vi "data to registers.vi"(9 "specifications":T1[](array[typedef]), 10 "allocation":u16[](array[numeric]), 11 "data table":T3) -> (2 "registers":u16[](array[numeric]), 3 "allocation":T3)   [LabVIEW 2013, in "Modbus Slave runtime.lvclass"]
uses:
  Modbus Slave runtime.lvclass
  <vilib>/NI/Tag Bus/table/data table.ctl
  data mapping elements.ctl
  <vilib>/NI/Tag Bus/tag/Data Type.ctl
  <vilib>/NI/Tag Bus/table/data polymorphs/read one/read Double.vi
  <vilib>/NI/Tag Bus/table/data polymorphs/read one/read Single.vi
  <vilib>/NI/Tag Bus/table/data polymorphs/read one/read I64.vi
  <vilib>/NI/Tag Bus/table/data polymorphs/read one/read U64.vi
  <vilib>/NI/Tag Bus/table/data polymorphs/read one/read I32.vi
  <vilib>/NI/Tag Bus/table/data polymorphs/read one/read U32.vi
  <vilib>/NI/Tag Bus/table/data polymorphs/read one/read I16.vi
  <vilib>/NI/Tag Bus/table/data polymorphs/read one/read U16.vi
  <vilib>/NI/Tag Bus/table/data polymorphs/read one/read I8.vi
  <vilib>/NI/Tag Bus/table/data polymorphs/read one/read U8.vi
  <vilib>/NI/Tag Bus/table/data polymorphs/read one/read Boolean.vi
  <vilib>/NI/Tag Bus/table/data table.lvlib
  <vilib>/NI/Tag Bus/tag/tag descriptor.lvclass
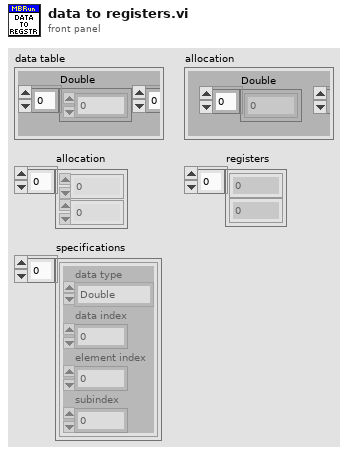
[diagram p1: front panel]
types:
  T1 = typedef "Modbus Slave runtime.lvclass/data mapping elements.ctl" = cluster{"data type":T2, "data index":i32, "element index":i32, "subindex":i32}
  T2 = typedef "tag bus.lvlib/tag descriptor.lvclass/Data Type.ctl" = enum16{"Double", "Single", "I64", "I32", "I16", "I8", "U64", "U32", "U16", "U8", "Boolean", "String", "Array of Double", "Array of Single", "Array of I64", "Array of I32", "Array of I16", "Array of I8", "Array of U64", "Array of U32", "Array of U16", "Array of U8", "Array of Boolean", "Array of String"}
  T3 = typedef "tag bus.lvlib/data table.lvlib/data table.ctl" = cluster{"Double":dbl[], "Single":sgl[], "I64":i64[], "I32":i32[], "I16":i16[], "I8":i8[], "U64":u64[], "U32":u32[], "U16":u16[], "U8":u8[], "Boolean":bool[], "String":string[], "Array of Double":cluster{"DBL Array":dbl[]}[], "Array of Single":cluster{"SGL Array":sgl[]}[], "Array of I64":cluster{"I64 Array":i64[]}[], "Array of I32":cluster{"I32 Array":i32[]}[], "Array of I16":cluster{"I16 Array":i16[]}[], "Array of I8":cluster{"I8 Array":i8[]}[], "Array of U64":cluster{"U64 Array":u64[]}[], "Array of U32":cluster{"U32 Array":u32[]}[], "Array of U16":cluster{"U16 Array":u16[]}[], "Array of U8":cluster{"U8 Array":u8[]}[], "Array of Boolean":cluster{"Boolean Array":bool[]}[], "Array of String":cluster{"String Array":string[]}[]}
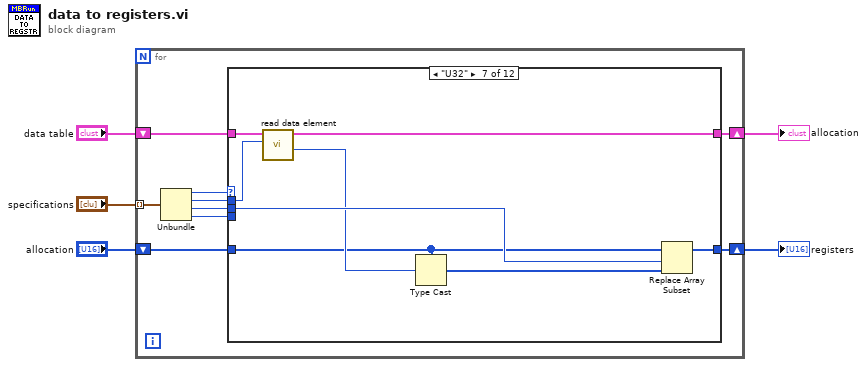
[diagram p0: block diagram]
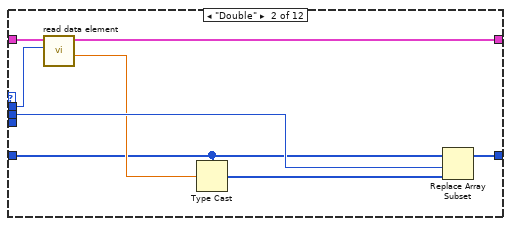
[diagram p3: hidden frame]
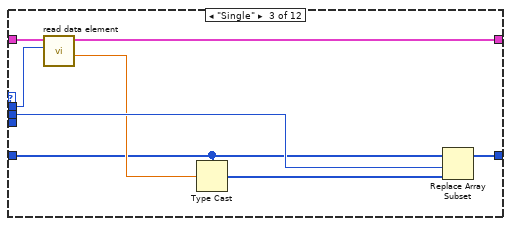
[diagram p4: hidden frame]
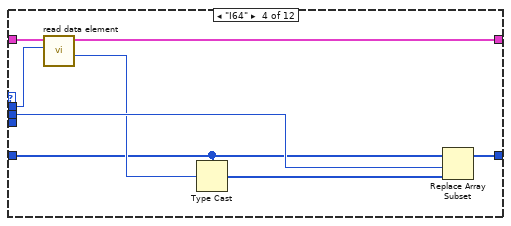
[diagram p5: hidden frame]
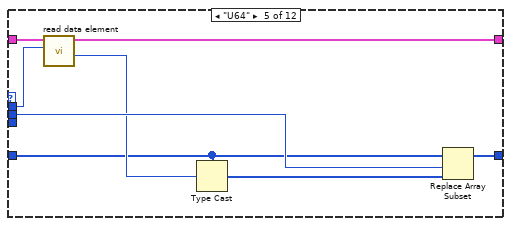
[diagram p6: hidden frame]
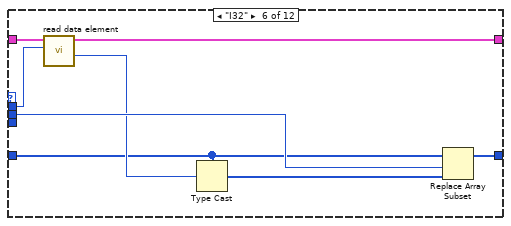
[diagram p7: hidden frame]
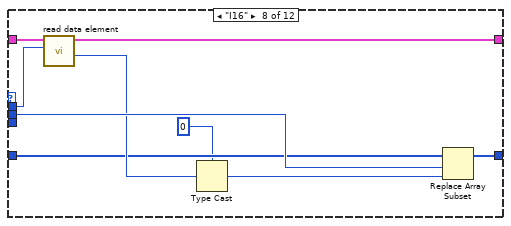
[diagram p8: hidden frame]
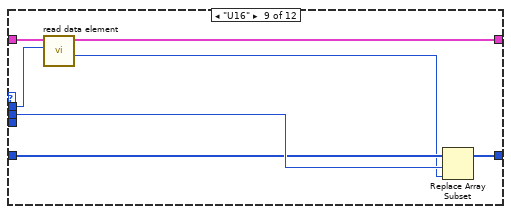
[diagram p9: hidden frame]
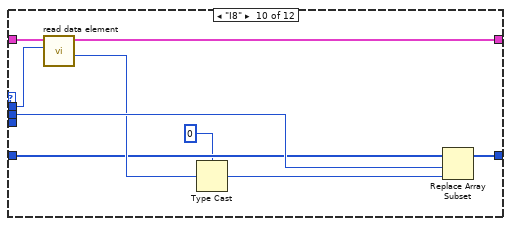
[diagram p10: hidden frame]
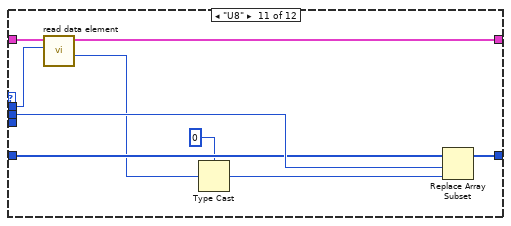
[diagram p11: hidden frame]
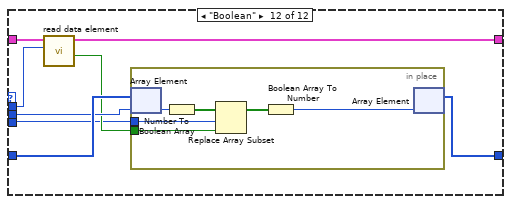
[diagram p12: hidden frame]
diagram:
  n1 = for {
    shift-right: [w11] -> w4
    shift-left: "data table" -> [w12]
    tunnel: "specifications" -> [w14] mode=indexing
    shift-right: [w7] -> w1
    shift-left: "allocation" -> [w10]
    n2 = Unbundle(w14) -> ("data type"=w13:T2, "data index"=w9:i32, "element index"=w6:i32, "subindex"=w8:i32)
    n3 = case shown="\"U32\"" w13 {
      tunnel: w12 -> [w16 w24 w32 w40 w48 w56 w64 w73 w80 w89 w98 w106]
      tunnel: [w16 w23 w31 w39 w47 w55 w63 w72 w79 w88 w97 w105] -> w11
      tunnel: w6 -> [_ w20 w28 w36 w44 w52 w60 w69 w76 w85 w94 w101]
      tunnel: w10 -> [w15 w18 w26 w34 w42 w50 w58 w67 w75 w83 w93 w103]
      tunnel: w9 -> [_ w22 w30 w38 w46 w54 w62 w71 w78 w87 w96 w104]
      tunnel: w8 -> [_ _ _ _ _ _ _ _ _ _ _ w99]
      tunnel: [w15 w21 w29 w37 w45 w53 w61 w70 w77 w86 w95 w102] -> w7
      frame Default {
      }
      frame "Double" {
        n4 = call-poly <vilib>:"read data element.vi"("index"=w22, "data table in"=w24) -> ("value"=w19:dbl, "data table out"=w23:T3)  [unwired: 8 in]
        n5 = Type Cast(type=w18, x=w19) -> (*(type *) &x=w17:u16[])
        n6 = Replace Array Subset(array=w18, new element=w17, index=w20) -> (w21:u16[])
      }
      frame "Single" {
        n7 = call-poly <vilib>:"read data element.vi"("index"=w30, "data table in"=w32) -> ("value"=w27:sgl, "data table out"=w31:T3)  [unwired: 8 in]
        n8 = Type Cast(type=w26, x=w27) -> (*(type *) &x=w25:u16[])
        n9 = Replace Array Subset(array=w26, new element=w25, index=w28) -> (w29:u16[])
      }
      frame "I64" {
        n10 = call-poly <vilib>:"read data element.vi"("index"=w38, "data table in"=w40) -> ("value"=w35:i64, "data table out"=w39:T3)  [unwired: 8 in]
        n11 = Type Cast(type=w34, x=w35) -> (*(type *) &x=w33:u16[])
        n12 = Replace Array Subset(array=w34, new element=w33, index=w36) -> (w37:u16[])
      }
      frame "U64" {
        n13 = call-poly <vilib>:"read data element.vi"("index"=w46, "data table in"=w48) -> ("value"=w43:u64, "data table out"=w47:T3)  [unwired: 8 in]
        n14 = Type Cast(type=w42, x=w43) -> (*(type *) &x=w41:u16[])
        n15 = Replace Array Subset(array=w42, new element=w41, index=w44) -> (w45:u16[])
      }
      frame "I32" {
        n16 = call-poly <vilib>:"read data element.vi"("index"=w54, "data table in"=w56) -> ("value"=w51:i32, "data table out"=w55:T3)  [unwired: 8 in]
        n17 = Type Cast(type=w50, x=w51) -> (*(type *) &x=w49:u16[])
        n18 = Replace Array Subset(array=w50, new element=w49, index=w52) -> (w53:u16[])
      }
      frame "U32" {
        n19 = call-poly <vilib>:"read data element.vi"("index"=w62, "data table in"=w64) -> ("value"=w59:u32, "data table out"=w63:T3)  [unwired: 8 in]
        n20 = Type Cast(type=w58, x=w59) -> (*(type *) &x=w57:u16[])
        n21 = Replace Array Subset(array=w58, new element=w57, index=w60) -> (w61:u16[])
      }
      frame "I16" {
        n22 = call-poly <vilib>:"read data element.vi"("index"=w71, "data table in"=w73) -> ("value"=w68:i16, "data table out"=w72:T3)  [unwired: 8 in]
        n23 = Type Cast(type=u16 0, x=w68) -> (*(type *) &x=w66:u16)
        n24 = Replace Array Subset(array=w67, new element=w66, index=w69) -> (w70:u16[])
      }
      frame "U16" {
        n25 = call-poly <vilib>:"read data element.vi"("index"=w78, "data table in"=w80) -> ("value"=w74:u16, "data table out"=w79:T3)  [unwired: 8 in]
        n26 = Replace Array Subset(array=w75, new element=w74, index=w76) -> (w77:u16[])
      }
      frame "I8" {
        n27 = call-poly <vilib>:"read data element.vi"("index"=w87, "data table in"=w89) -> ("value"=w84:i8, "data table out"=w88:T3)  [unwired: 8 in]
        n28 = Type Cast(type=u16 0, x=w84) -> (*(type *) &x=w82:u16)
        n29 = Replace Array Subset(array=w83, new element=w82, index=w85) -> (w86:u16[])
      }
      frame "U8" {
        n30 = call-poly <vilib>:"read data element.vi"("index"=w96, "data table in"=w98) -> ("value"=w92:u8, "data table out"=w97:T3)  [unwired: 8 in]
        n31 = Type Cast(type=u16 0, x=w92) -> (*(type *) &x=w91:u16)
        n32 = Replace Array Subset(array=w93, new element=w91, index=w94) -> (w95:u16[])
      }
      frame "Boolean" {
        n33 = call-poly <vilib>:"read data element.vi"("index"=w104, "data table in"=w106) -> ("value"=w100:bool, "data table out"=w105:T3)  [unwired: 8 in]
        n34 = in-place {
          in-place-border: w100 -> [w108]
          in-place-border: w99 -> [w107]
          n35 = in-place-array #1(w103, w101) -> (w112:u16)
          n36 = Number To Boolean Array(number=w112) -> (Boolean array=w110:bool[])
          n37 = Replace Array Subset(array=w110, new element=w108, index=w107) -> (w109:bool[])
          n38 = Boolean Array To Number(Boolean array=w109) -> (number=w111:u16)
          n39 = in-place-array #1(w111) -> (w102:u16[])  [unwired: 1 out]
        }
      }
    }
  }
  "allocation" <- w4
  "registers" <- w1
